vi "Get Frame Timestamp.vi"(0 "error in (no error)":errorcluster, 1 "Input Image":T1) -> (2 "error out":errorcluster, 3 "System Time Stamp":timestamp, 4 "Output Image":T1(plugin-control))   [LabVIEW 2014]
uses:
  <vilib>/vision/Image Controls.llb/IMAQ Image.ctl
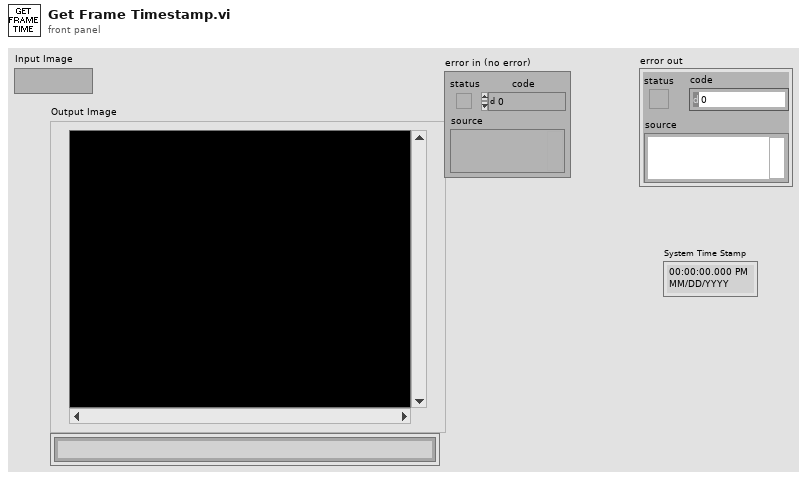
[diagram p1: front panel]
types:
  T1 = typedef "IMAQ Image.ctl" = refnum<image>
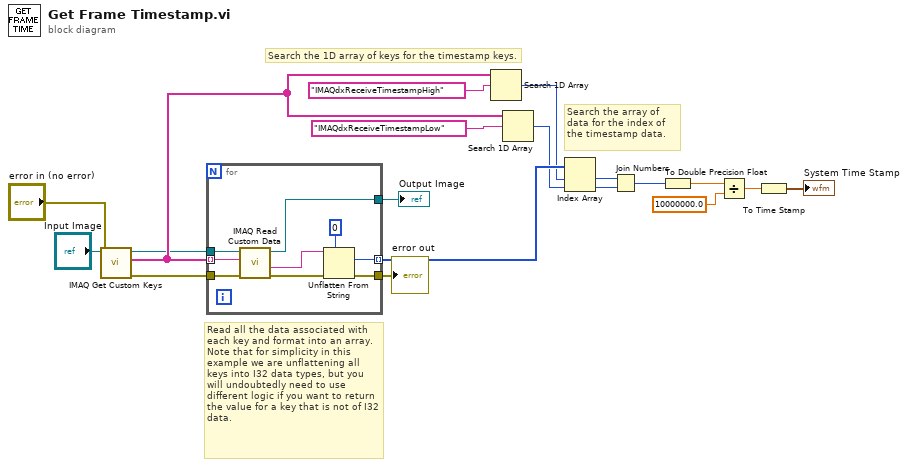
[diagram p0: block diagram]
diagram:
  # "Search the array of data for the index of the timestamp data."
  # "Search the 1D array of keys for the timestamp keys."
  # "Read all the data associated with each key and format into an array. Note that for simplicity in this example we are unflattening all keys into I32 data types, but you will undoubtedly need to use different logic if you want to return the value for a key that is not of I32 data."
  n1 = call "IMAQ Get Custom Keys"("error in (no error)"="error in (no error)", "Image"="Input Image") -> ("error out"=w19:errorcluster, "Keys"=w13:string[], "Image (duplicate)"=w5:T1)  [unwired: 6 in, 1 out]
  n2 = for {
    tunnel: w5 -> [w28]
    tunnel: w19 -> [w27]
    tunnel: [w26] -> w2
    tunnel: w13 -> [w24] mode=indexing
    tunnel: [w25] -> w4
    tunnel: [w23] -> w18 mode=indexing
    n3 = call "IMAQ Read Custom Data"("error in (no error)"=w27, "Key"=w24, "Image"=w28) -> ("error out"=w22:errorcluster, "Custom Data Out"=w21:string, "Image (duplicate)"=w25:T1)  [unwired: 6 in]
    n4 = Unflatten From String(type=0, binary string=w21, error in (no error)=w22) -> (value=w23:i32, error out=w26:errorcluster)  [unwired: 2 in, 1 out]
  }
  "Output Image" <- w4
  "error out" <- w2
  n5 = Search 1D Array(1D array=w13, element="IMAQdxReceiveTimestampHigh") -> (index of element=w14:i32)  [unwired: 1 in]
  n6 = Search 1D Array(1D array=w13, element="IMAQdxReceiveTimestampLow") -> (index of element=w15:i32)  [unwired: 1 in]
  n7 = Index Array(array=w18, index #1=w14, index #2=w15) -> (element #1=w11:i32, element #2=w12:i32)
  n8 = Join Numbers(hi=w11, lo=w12) -> ((hi.lo)=w10:u64)
  n9 = To Double Precision Float(number=w10) -> (double precision float=w9:dbl)
  n10 = Divide(x=w9, y=10000000.0) -> (x/y=w7:dbl)
  n11 = To Time Stamp(1:w7) -> (0:→"System Time Stamp":timestamp)
